vi "Msg to Send.vi"(10 "Error":errorcluster) -> (3 "LVCAM Destroy Self Msg out":refnum<class "LVCAM Destroy Self Msg.lvclass">)   [LabVIEW 2021, in "LVCAM Destroy Self.lvlib" / "LVCAM Destroy Self Msg.lvclass"]
uses:
  LVCAM Destroy Self Msg.lvclass
  LVCAM Destroy Self Msg.lvclass/LVCAM Destroy Self Msg.ctl
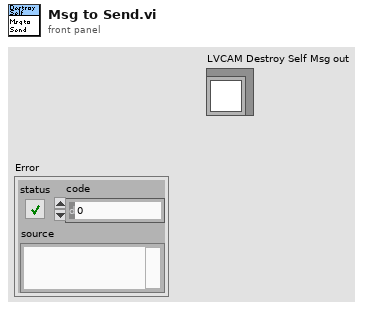
[diagram p1: front panel]
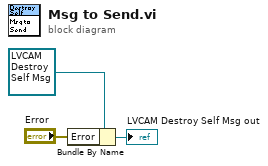
[diagram p0: block diagram]
diagram:
  n1 = Bundle By Name(cluster=refnum<class "LVCAM Destroy Self Msg.lvclass"> refnum ("Destroy Msg in"), "Error"="Error") -> (→"LVCAM Destroy Self Msg out":refnum<class "LVCAM Destroy Self Msg.lvclass">)
